vi "configure timestamp delay.vi"(7 "delay":u16, 8 "error in (no error)":errorcluster, 9 "ckpulses":u16, 10 "Board":u16, 11 "identifier":string) -> (0 "error out":errorcluster, 3 "function return":u32)   [LabVIEW 2015, in "XGL_DPP.lvlib"]
doc: "EXTERN DECLSPEC uint32_t CALL_CONV configure_timestamp_delay(const char * identifier, uint16_t Board, uint16_t ckpulses, uint16_t delay);"
uses:
  XGL_DPP.lvlib
  XGL_DPP.dll
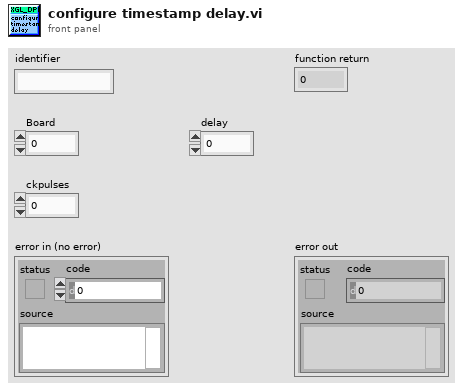
[diagram p1: front panel]
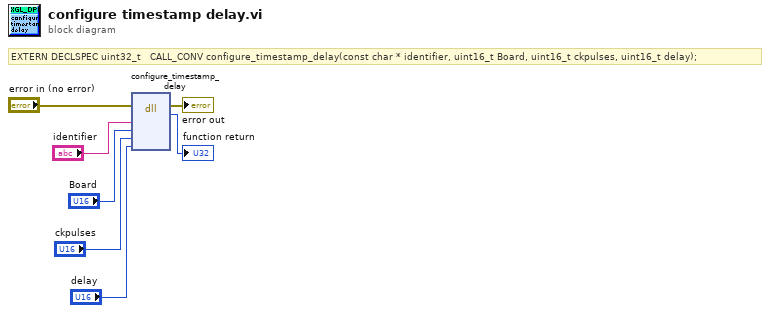
[diagram p0: block diagram]
diagram:
  # "EXTERN DECLSPEC uint32_t   CALL_CONV configure_timestamp_delay(const char * identifier, uint16_t Board, uint16_t ckpulses, uint16_t delay);"
  n1 = dll-call lib="D:/Users/XRF/Desktop/Scanning Software_Demokritos_2015_v7/libs/Vis_2/XGL_DPP.*" fn="configure_timestamp_delay"(error in="error in (no error)", "identifier"="identifier", "Board"="Board", "ckpulses"="ckpulses", "delay"="delay") -> (error out=→"error out":errorcluster, →"function return":u32)  [unwired: 6 in, 1 out]
